vi "locate channel.vi"(10 "tag descriptor":refnum<class "tag descriptor.lvclass">, 11 "sequencer config in":refnum<class "base TBM sequencer configuration.lvclass">) -> (2 "index":i32, 3 "sequencer config out":refnum<class "base TBM sequencer configuration.lvclass">)   [LabVIEW 2014, in "base TBM sequencer configuration.lvclass"]
uses:
  base TBM sequencer configuration.lvclass
  <vilib>/NI/Tag Bus/tag/tag descriptor.lvclass
  base TBM sequencer configuration.lvclass/base TBM sequencer configuration.ctl
  <vilib>/NI/Tag Bus/tag/tag descriptor.lvclass/tag descriptor.ctl
  <vilib>/NI/Tag Bus/tag/read tag name.vi
  <vilib>/NI/Tag Bus Module Framework/channel/TBM channel.lvclass
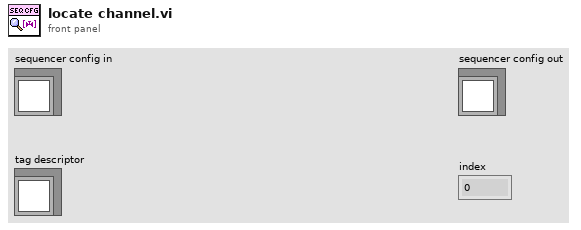
[diagram p1: front panel]
types:
  T1 = typedef "base TBM sequencer configuration.lvclass/Tag Info.ctl" = cluster{"Channel":refnum<class "TBM channel.lvclass">, "Writers":string[], "Readers":string[], "Owning ID":string}
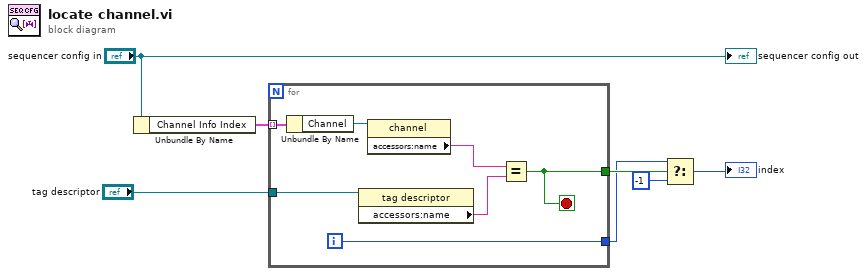
[diagram p0: block diagram]
diagram:
  n1 = Unbundle By Name("sequencer config in") -> ("Channel Info Index"=w5:T1[])
  n2 = for {
    tunnel: "tag descriptor" -> [w14]
    tunnel: w5 -> [w8] mode=indexing
    tunnel: [w11] -> w4
    tunnel: [w10] -> w3
    i -> [w10]
    stop <- w11 stop-if-true
    n3 = Unbundle By Name(w8) -> ("Channel"=w9:refnum<class "TBM channel.lvclass">)
    n4 = property class="tag descriptor"(reference=w14) -> ("accessors:name"=w12:string)  [unwired: 1 in, 2 out]
    n5 = property class="channel"(reference=w9) -> ("accessors:name"=w13:string)  [unwired: 1 in, 2 out]
    n6 = Equal?(x=w13, y=w12) -> (x = y?=w11:bool)
  }
  n7 = Select(t=w3, s=w4, f=-1) -> (s? t:f=→"index":i32)
  "sequencer config out" <- "sequencer config in"
